vi "Settings.vi"(8 "error in (no error)":errorcluster) -> (0 "error out":errorcluster)   [LabVIEW 2013]
uses:
  Anemometry Sub Vis/Globals/Constants_global.vi
  <vilib>/Utility/config.llb/Read Key (Path).vi
  <vilib>/Utility/config.llb/NI_LVConfig.lvlib
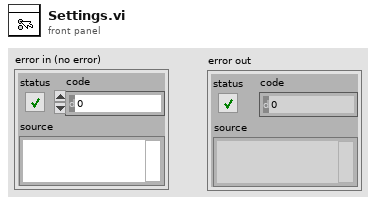
[diagram p1: front panel]
types:
  T1 = enum32{"invalid app kind", "Development System", "Run Time System", "Student Edition", "Embedded LabVIEW", "Evaluation", "Custom"}
  T2 = typedef "NI_LVConfig.lvlib/Config Data RefNum.ctl" = refnum<k1>
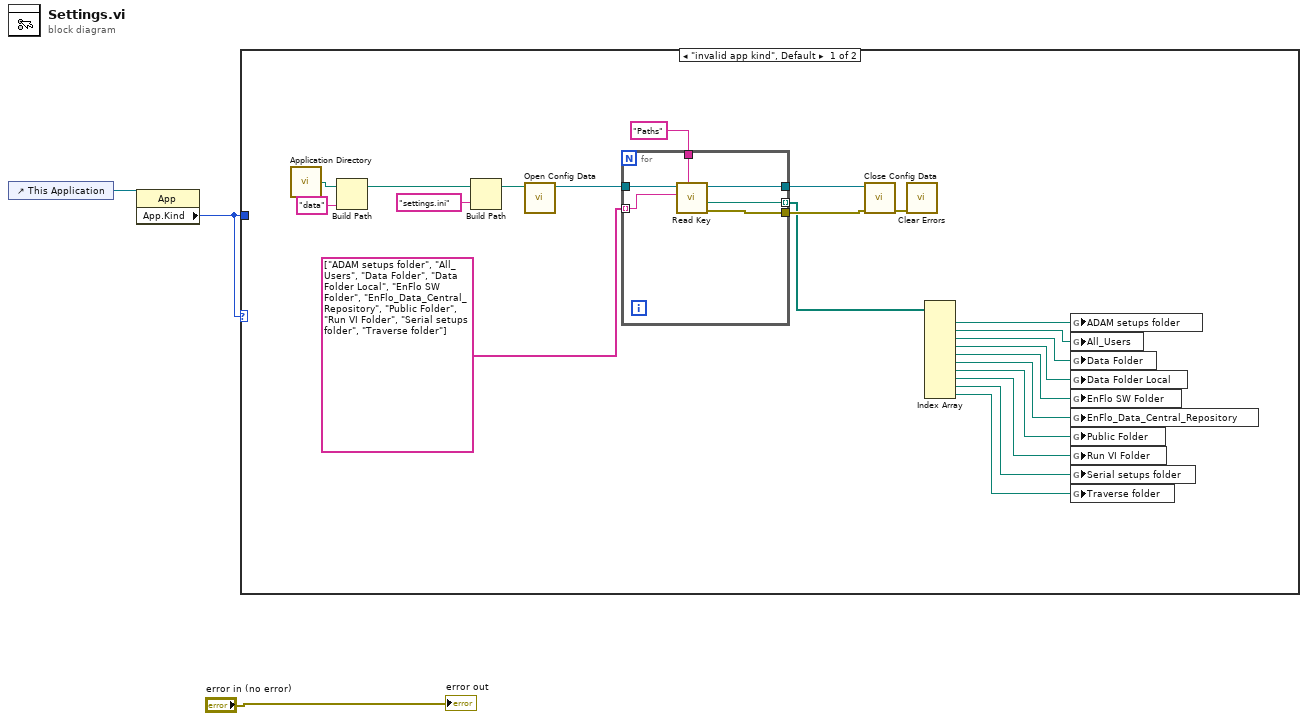
[diagram p0: block diagram]
diagram:
  n1 = control-ref of="This Application"() -> (w3:refnum<vi>)
  n2 = property class="App"(reference=w3) -> ("App.Kind"=w1:T1)  [unwired: 1 in, 2 out]
  n3 = case shown="\"invalid app kind\", Default" w1 {
    tunnel: w1 -> [_ _]
    frame "invalid app kind", Default {
      n4 = call <vilib>:"Application Directory.vi"() -> ("Application Directory"=w5:path)
      n5 = Build Path(base path=w5, name or relative path="data") -> (appended path=w25:path)
      n6 = Build Path(base path=w25, name or relative path="settings.ini") -> (appended path=w24:path)
      n7 = call <vilib>:"Open Config Data.vi"("configuration file path"=w24) -> ("refnum"=w22:T2)  [unwired: 8 in, 2 out]
      n8 = for {
        tunnel: w22 -> [w31]
        tunnel: "Paths" ("section") -> [w30]
        tunnel: string[] ["ADAM setups folder", "All_Users", "Data Folder", "Data Folder Local", "EnFlo SW Folder", "EnFlo_Data_Central_Repository", "Public Folder", "Run VI Folder", "Serial setups folder", "Traverse folder"] -> [w29] mode=indexing
        tunnel: [w28] -> w16 mode=indexing
        tunnel: [w27] -> w19
        tunnel: [w26] -> w18
        n9 = call-poly <vilib>:"Read Key.vi"("section"=w30, "key"=w29, "refnum"=w31) -> ("error out"=w26:errorcluster, "value"=w28:path, "refnum out"=w27:T2)  [unwired: 5 in, 1 out]
      }
      n10 = call <vilib>:"Close Config Data.vi"("error in (no error)"=w18, "refnum"=w19) -> ("error out"=w17:errorcluster)  [unwired: 8 in, 1 out]
      n11 = call <vilib>:"Clear Errors.vi"("error in (no error)"=w17) -> ()  [unwired: 6 in, 1 out]
      n12 = Index Array(array=w16) -> (element #1=w15:path, element #2=w14:path, element #3=w13:path, element #4=w12:path, element #5=w11:path, element #6=w10:path, element #7=w9:path, element #8=w8:path, element #9=w7:path, element #10=w6:path)  [unwired: 10 in]
      n13 = global write "Constants_global.vi" "ADAM setups folder"(w15) -> ()
      n14 = global write "Constants_global.vi" "All_Users"(w14) -> ()
      n15 = global write "Constants_global.vi" "Data Folder"(w13) -> ()
      n16 = global write "Constants_global.vi" "Data Folder Local"(w12) -> ()
      n17 = global write "Constants_global.vi" "EnFlo SW Folder"(w11) -> ()
      n18 = global write "Constants_global.vi" "EnFlo_Data_Central_Repository"(w10) -> ()
      n19 = global write "Constants_global.vi" "Public Folder"(w9) -> ()
      n20 = global write "Constants_global.vi" "Run VI Folder"(w8) -> ()
      n21 = global write "Constants_global.vi" "Serial setups folder"(w7) -> ()
      n22 = global write "Constants_global.vi" "Traverse folder"(w6) -> ()
    }
    frame "Development System" {
    }
  }
  "error out" <- "error in (no error)"
